vi "Read Cancel build ref.vi"(11 "SolutionBuilder in":refnum<class "SolutionBuilder.lvclass">) -> (2 "Cancel build ref":refnum<vi>, 3 "SolutionBuilder out":refnum<class "SolutionBuilder.lvclass">)   [LabVIEW 2019, in "SolutionBuilder.lvlib" / "SolutionBuilder.lvclass"]
uses:
  SolutionBuilder.lvclass
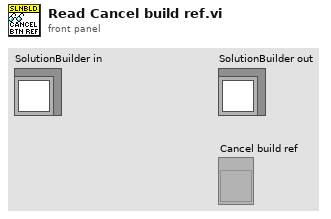
[diagram p1: front panel]
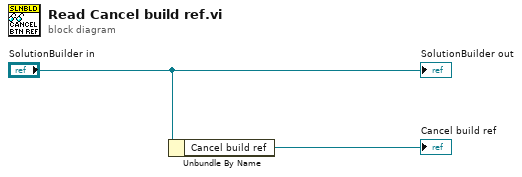
[diagram p0: block diagram]
diagram:
  n1 = Unbundle By Name("SolutionBuilder in") -> ("Cancel build ref"=→"Cancel build ref":refnum<vi>)
  "SolutionBuilder out" <- "SolutionBuilder in"
